vi "getVideo.vi"(8 "error in (no error)":errorcluster, 10 "Video Id":string, 11 "ThirdPartyYoutubeClass in":refnum<class "ThirdPartyYoutubeClass.lvclass">) -> (0 "error out":errorcluster, 2 "Video":refnum<class "Video.lvclass">, 3 "ThirdPartyYoutubeClass out":refnum<class "ThirdPartyYoutubeClass.lvclass">)   [LabVIEW 2017, in "ThirdPartyYoutubeClass.lvclass"]
uses:
  ThirdPartyYoutubeClass.lvclass
  Video Class/Video.lvclass
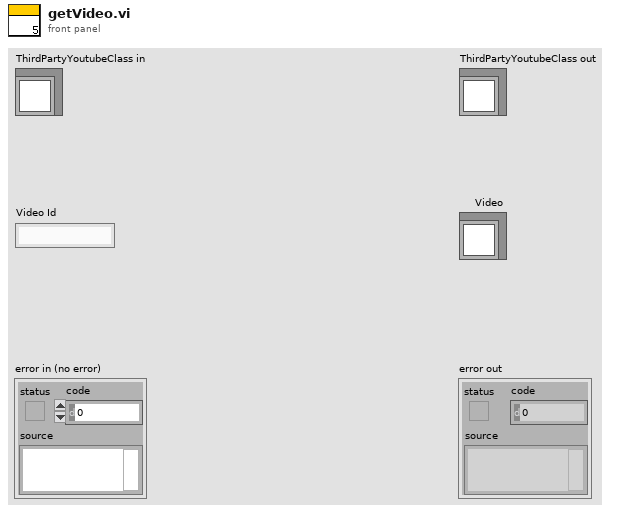
[diagram p1: front panel]
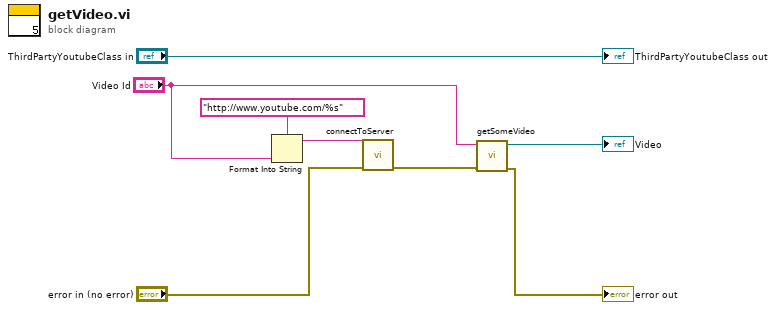
[diagram p0: block diagram]
diagram:
  n1 = Format Into String(format string="http://www.youtube.com/%s" ("string"), "Video Id") -> (resulting string=w4:string)  [unwired: 2 in, 1 out]
  n2 = call "connectToServer.vi"("error in (no error)"="error in (no error)", "server"=w4) -> ("error out"=w5:errorcluster)  [unwired: 9 in]
  n3 = call "getSomeVideo.vi"("error in (no error)"=w5, "videoId"="Video Id") -> ("error out"=→"error out":errorcluster, "Video out"=→"Video":refnum<class "Video.lvclass">)  [unwired: 8 in]
  "ThirdPartyYoutubeClass out" <- "ThirdPartyYoutubeClass in"
